vi "init2D.vi"(7 "B [T]":dbl=1.0, 10 "calib(pixel) out out":T1, 11 "Cam out":T2) -> (1 "2D":T8, 2 "calib(pixel) out out 2":T1, 3 "Cam out 2":T2)   [LabVIEW 2020]
uses:
  calibPixel.ctl
  CamSettingSUB_TypDEf.ctl
  MagAnalysis_Online_Bella/SubVis/CamAndObj_TypDEf.ctl
  shared/OnOffTypeDef.ctl
  userROI.ctl
  shared/numericVariable_TypeDef.ctl
  CamRoiTypDef.ctl
  2DTypDef.ctl
  BaseDriver/BaseDriver.lvclass
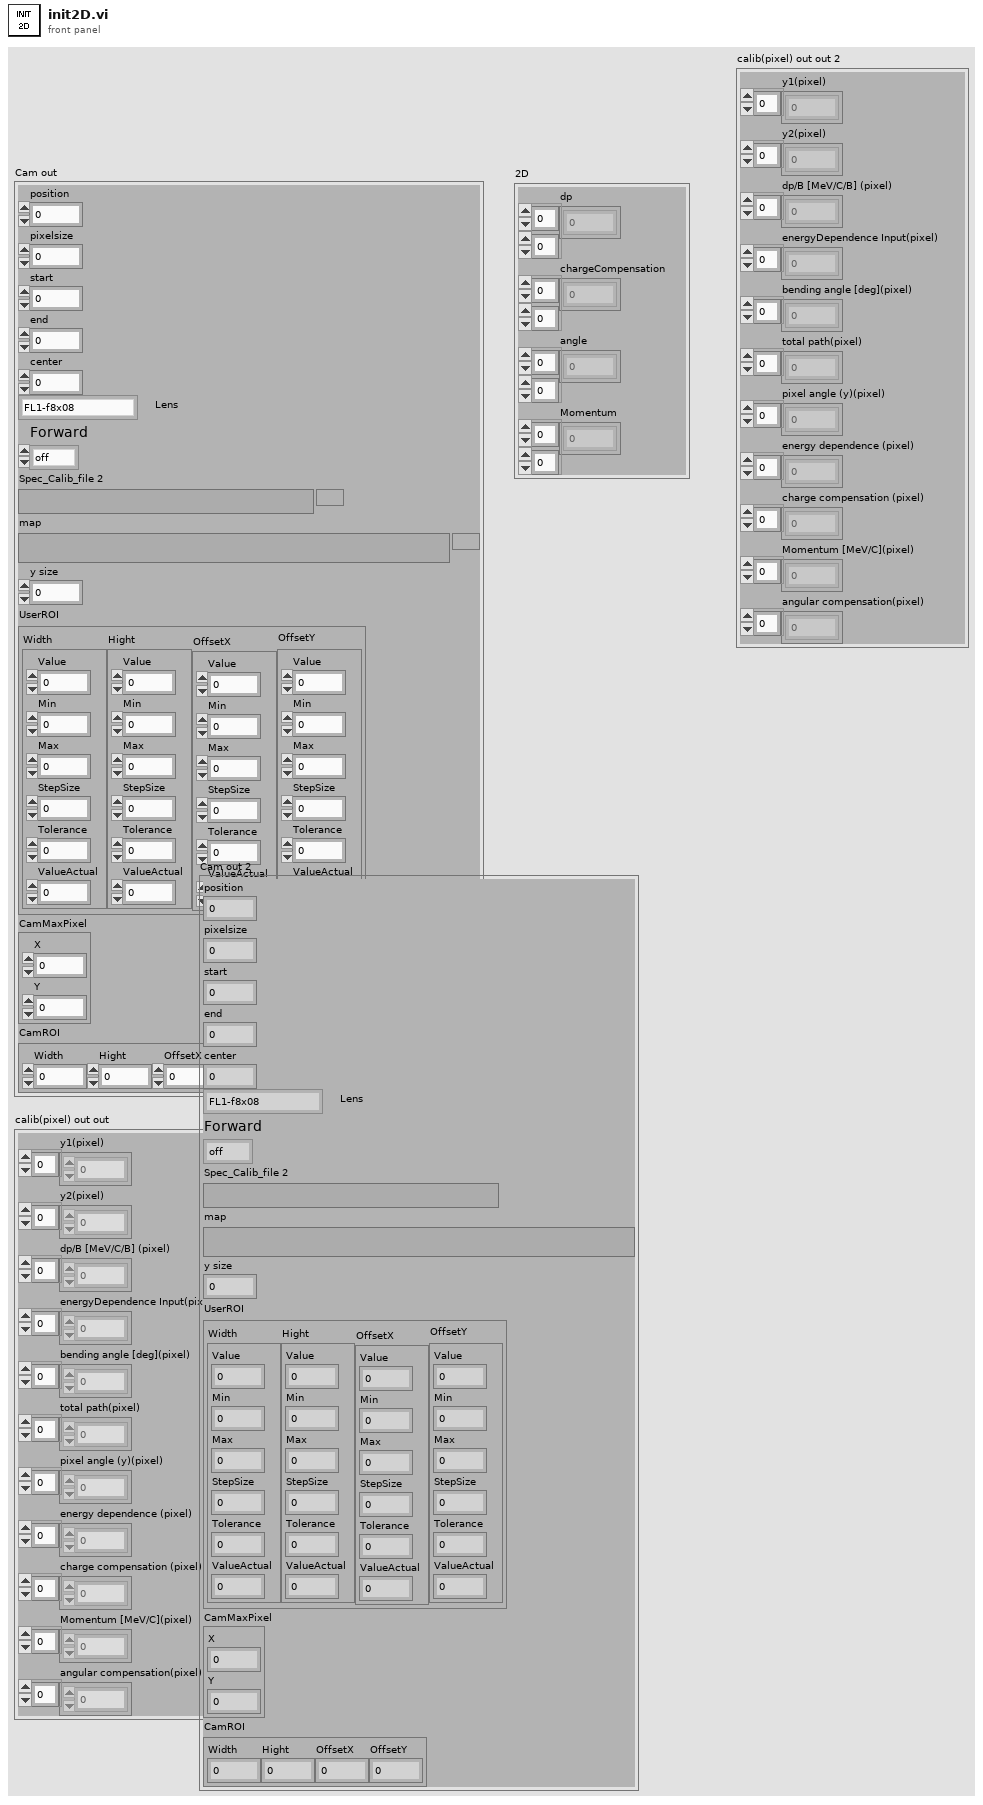
[diagram p1: front panel]
types:
  T1 = typedef "calibPixel.ctl" = cluster{"y1(pixel)":dbl[], "y2(pixel)":dbl[], "dp/B [MeV/C/B] (pixel)":dbl[], "energyDependence Input(pixel)":dbl[], "bending angle [deg](pixel)":dbl[], "total path(pixel)":dbl[], "pixel angle (y)(pixel)":dbl[], "energy dependence (pixel)":dbl[], "charge compensation (pixel)":dbl[], "Momentum [MeV/C](pixel)":dbl[], "angular compensation(pixel)":dbl[]}
  T2 = typedef "CamSettingSUB_TypDEf.ctl" = cluster{"position":dbl, "pixelsize":dbl, "start":dbl, "end":dbl, "center":dbl, "Lens":T3, "Forward":T4, "Spec_Calib_file 2":path, "map":path, "y size":i32, "UserROI":T5, "CamMaxPixel":cluster{"X":i32, "Y":i32}, "CamROI":T7}
  T3 = typedef "CamAndObj_TypDEf.ctl" = enum16{"FL1-f8x08", "FL1-f8x06", "FL1-f8", "ch300-f50", "FL2G-f8", "FL3M14-f8", "FL3M14-f8x08", "FL3M14-f8x08(2x2)"}
  T4 = typedef "OnOffTypeDef.ctl" = enum16{"off", "on"}
  T5 = typedef "userROI.ctl" = cluster{"Width":T6, "Hight":T6, "OffsetX":T6, "OffsetY":T6}
  T6 = typedef "BaseDriver.lvclass/numericVariable_TypeDef.ctl" = cluster{"Value":dbl, "Min":dbl, "Max":dbl, "StepSize":dbl, "Tolerance":dbl, "ValueActual":dbl}
  T7 = typedef "CamRoiTypDef.ctl" = cluster{"Width":dbl, "Hight":dbl, "OffsetX":dbl, "OffsetY":dbl}
  T8 = typedef "2DTypDef.ctl" = cluster{"dp":dbl[][], "chargeCompensation":dbl[][], "angle":dbl[][], "Momentum":dbl[][]}
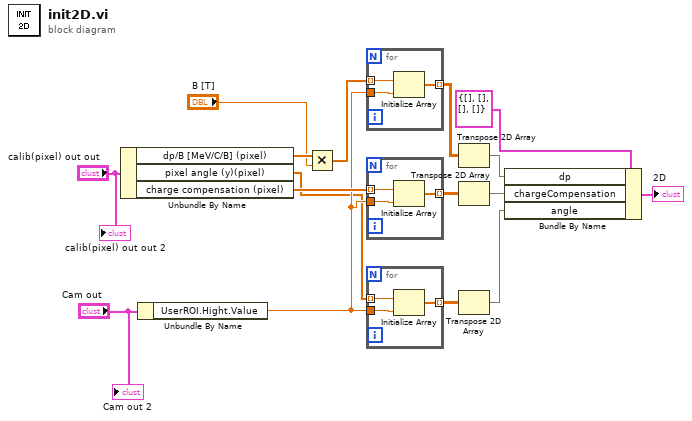
[diagram p0: block diagram]
diagram:
  n1 = Unbundle By Name("calib(pixel) out out") -> ("dp/B [MeV/C/B] (pixel)"=w12:dbl[], "pixel angle (y)(pixel)"=w6:dbl[], "charge compensation (pixel)"=w14:dbl[])
  n2 = Unbundle By Name("Cam out") -> ("UserROI.Hight.Value"=w13:dbl)
  n3 = Multiply(x=w12, y="B [T]") -> (x*y=w4:dbl[])
  n4 = for {
    tunnel: w4 -> [w19] mode=indexing
    tunnel: [w18] -> w3 mode=indexing
    tunnel: w13 -> [w17]
    n5 = Initialize Array(w19, w17) -> (w18:dbl[])
  }
  n6 = for {
    tunnel: w14 -> [w22] mode=indexing
    tunnel: [w21] -> w5 mode=indexing
    tunnel: w13 -> [w20]
    n7 = Initialize Array(w22, w20) -> (w21:dbl[])
  }
  n8 = for {
    tunnel: w6 -> [w25] mode=indexing
    tunnel: [w24] -> w2 mode=indexing
    tunnel: w13 -> [w23]
    n9 = Initialize Array(w25, w23) -> (w24:dbl[])
  }
  n10 = Transpose 2D Array(2D array=w3) -> (transposed array=w8:dbl[][])
  n11 = Transpose 2D Array(2D array=w5) -> (transposed array=w10:dbl[][])
  n12 = Transpose 2D Array(2D array=w2) -> (transposed array=w9:dbl[][])
  n13 = Bundle By Name(cluster=T8 {"dp"=[], "chargeCompensation"=[], "angle"=[], "Momentum"=[]} ("2D"), "dp"=w8, "chargeCompensation"=w10, "angle"=w9) -> (→"2D":T8)
  "Cam out 2" <- "Cam out"
  "calib(pixel) out out 2" <- "calib(pixel) out out"
